vi "Configure Multi Eval Meas List Segment PUSCH Allocation.vi"(0 "VISA resource name":refnum<visa-resource-name>, 1 "Allocation (1)":T1=1, 2 "No Symbols (4)":i32=4, 3 "No RBs (1)":i32=1, 5 "Instance (1)":T4=1, 7 "Segment (1)":T3=1, 9 "Carrier Component (1)":T2=1, 10 "Modulation Scheme (Pi/2-BPSK)":i32(ring) items=["Pi/2-BPSK", "QPSK", "16-QAM", "64-QAM", "256-QAM"], 11 "error in (no error)":errorcluster, 12 "Mapping Type (A)":i32(ring) items=["A", "B"], 13 "Start Symbol (0)":i32, 14 "Start RB (0)":i32) -> (4 "VISA resource name out":refnum<visa-resource-name>, 15 "error out":errorcluster)   [LabVIEW 2015, in "Rohde&Schwarz CMXP NR FR2 Measurement.lvlib"]
doc: "Specifies settings related to the PUSCH allocation, for carrier <cc>, allocation <a> in segment <no>.\n\nAttribute:\nRSCMXPNRFR2M_ATTR_MULTI_EVAL_MEASUREMENT_LIST_SEGMENT_PUSCH_ALLOCATION\n\nRemote-control command:\nCONFigure:NRMMw:MEAS<i>:LIST:SEGMent<no>[:CC<cc>]:ALLocation<a>:PUSCh"
uses:
  <instrlib>/Rohde&Schwarz CMXP NR FR2 Measurement/Rohde&Schwarz CMXP NR FR2 Measurement.lvlib
  <instrlib>/Rohde&Schwarz CMXP NR FR2 Measurement/Private/_Instance.ctl
  <instrlib>/Rohde&Schwarz CMXP NR FR2 Measurement/Private/_Segment.ctl
  <instrlib>/Rohde&Schwarz CMXP NR FR2 Measurement/Private/_Carrier Component.ctl
  <instrlib>/Rohde&Schwarz CMXP NR FR2 Measurement/Private/_Allocation.ctl
  <instrlib>/Rohde&Schwarz CMXP NR FR2 Measurement/Private/rsidr_core.llb/rsidr_core.lvlib
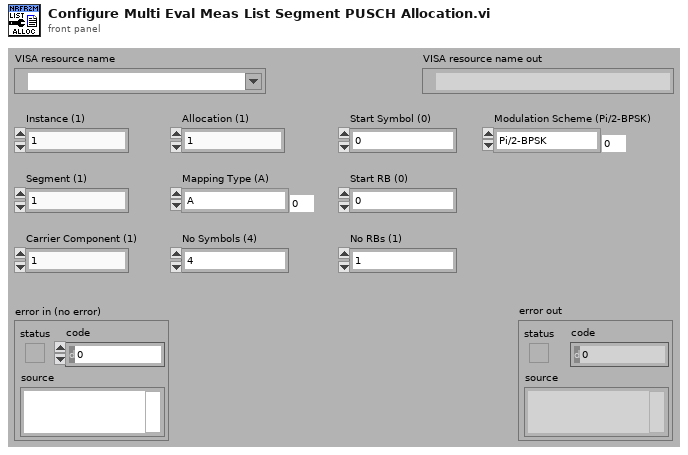
[diagram p1: front panel]
types:
  T1 = typedef "Rohde&Schwarz CMXP NR FR2 Measurement.lvlib/_Allocation.ctl" = i32
  T2 = typedef "Rohde&Schwarz CMXP NR FR2 Measurement.lvlib/_Carrier Component.ctl" = i32
  T3 = typedef "Rohde&Schwarz CMXP NR FR2 Measurement.lvlib/_Segment.ctl" = i32
  T4 = typedef "Rohde&Schwarz CMXP NR FR2 Measurement.lvlib/_Instance.ctl" = i32
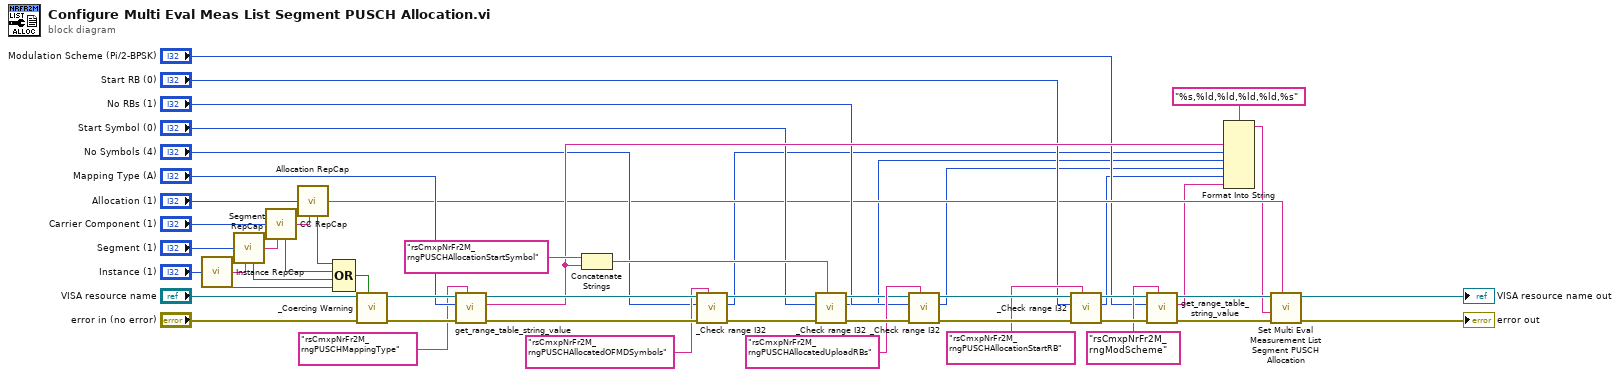
[diagram p0: block diagram]
diagram:
  n1 = call <instrlib>:"Instance RepCap.vi"("Instance In"="Instance (1)") -> ("In Range?"=w46:bool, "RepCap Identifier Out"=w2:string)  [unwired: 1 in]
  n2 = call <instrlib>:"Segment RepCap.vi"("Segment In"="Segment (1)", "RepCap String In (\"\")"=w2) -> ("In Range?"=w45:bool, "RepCap Identifier Out"=w44:string)
  n3 = call <instrlib>:"CC RepCap.vi"("CC In"="Carrier Component (1)", "RepCap String In (\"\")"=w44) -> ("In Range?"=w43:bool, "RepCap Identifier Out"=w42:string)
  n4 = call <instrlib>:"Allocation RepCap.vi"("Allocation In"="Allocation (1)", "RepCap String In (\"\")"=w42) -> ("In Range?"=w41:bool, "RepCap Identifier Out"=w10:string)
  n5 = Compound Arithmetic op=OR(w41, w43, w45, w46) -> (w48:bool)
  n6 = call <instrlib>:"_Coercing Warning.vi"("In Range?"=w48, "error in (no error)"="error in (no error)", "VISA resource name"="VISA resource name") -> ("error out"=w22:errorcluster, "VISA resource name out"=w23:refnum<visa-resource-name>)  [unwired: 7 in]
  n7 = call <instrlib>:"get_range_table_string_value.vi"("Range Table ID in"="rsCmxpNrFr2M_rngPUSCHMappingType", "error in"=w22, "I32 input"="Mapping Type (A)", "VISA resource name"=w23) -> ("error out"=w40:errorcluster, "String Value out"=w24:string, "VISA resource name out"=w39:refnum<visa-resource-name>)  [unwired: 5 in]
  n8 = Concatenate Strings("rsCmxpNrFr2M_rngPUSCHAllocationStartSymbol", w24) -> (w34:string)
  n9 = call <instrlib>:"_Check range I32.vi"("Range Table Identifier"="rsCmxpNrFr2M_rngPUSCHAllocatedOFMDSymbols", "error in (no error)"=w40, "I32 Value In"="No Symbols (4)", "VISA resource name"=w39) -> ("error out"=w37:errorcluster, "I32 Value Out"=w7:i32, "VISA resource name out"=w36:refnum<visa-resource-name>)  [unwired: 5 in]
  n10 = call <instrlib>:"_Check range I32.vi"("Range Table Identifier"=w34, "error in (no error)"=w37, "I32 Value In"="Start Symbol (0)", "VISA resource name"=w36) -> ("error out"=w33:errorcluster, "I32 Value Out"=w6:i32, "VISA resource name out"=w31:refnum<visa-resource-name>)  [unwired: 5 in]
  n11 = call <instrlib>:"_Check range I32.vi"("Range Table Identifier"="rsCmxpNrFr2M_rngPUSCHAllocatedUploadRBs", "error in (no error)"=w33, "I32 Value In"="No RBs (1)", "VISA resource name"=w31) -> ("error out"=w30:errorcluster, "I32 Value Out"=w5:i32, "VISA resource name out"=w29:refnum<visa-resource-name>)  [unwired: 5 in]
  n12 = call <instrlib>:"_Check range I32.vi"("Range Table Identifier"="rsCmxpNrFr2M_rngPUSCHAllocationStartRB", "error in (no error)"=w30, "I32 Value In"="Start RB (0)", "VISA resource name"=w29) -> ("error out"=w28:errorcluster, "I32 Value Out"=w4:i32, "VISA resource name out"=w27:refnum<visa-resource-name>)  [unwired: 5 in]
  n13 = call <instrlib>:"get_range_table_string_value.vi"("Range Table ID in"="rsCmxpNrFr2M_rngModScheme", "error in"=w28, "I32 input"="Modulation Scheme (Pi/2-BPSK)", "VISA resource name"=w27) -> ("error out"=w14:errorcluster, "String Value out"=w3:string, "VISA resource name out"=w15:refnum<visa-resource-name>)  [unwired: 5 in]
  n14 = Format Into String(format string="%s,%ld,%ld,%ld,%ld,%s", w24, w7, w6, w5, w4, w3) -> (resulting string=w1:string)  [unwired: 2 in, 1 out]
  n15 = call "Set Multi Eval Measurement List Segment PUSCH Allocation"("Repeated Capabilities"=w10, "error in (no error)"=w14, "Multi Eval Measurement List Segment PUSCH Allocation ()"=w1, "instrument handle"=w15) -> ("error out"=→"error out":errorcluster, "instrument handle out"=→"VISA resource name out":refnum<visa-resource-name>)  [unwired: 6 in]
